vi "TEST - String to Character Array.vi"(8 "error in (no error)":errorcluster) -> (0 "error out":errorcluster, 2 "Pass":bool)   [LabVIEW 2009]
panel:
  out "Expected Result":string[](array[string])
  out "Result":string[](array[string])
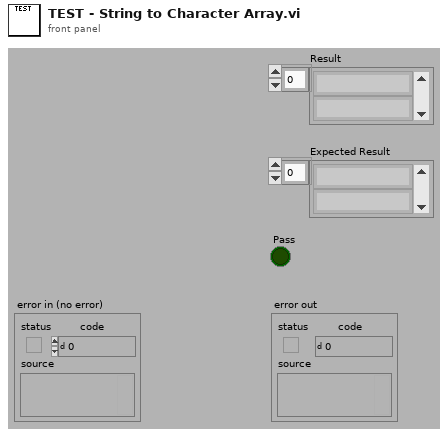
[diagram p1: front panel]
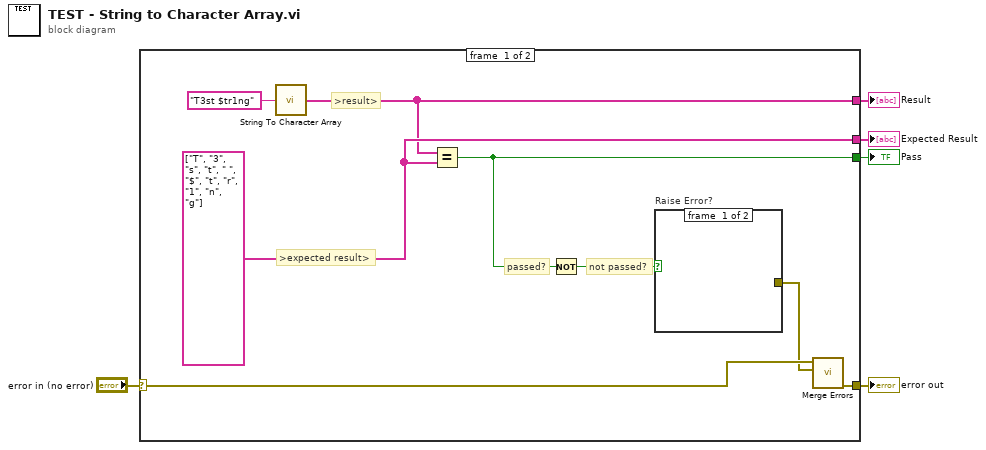
[diagram p0: block diagram]
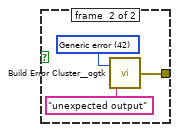
[diagram p2: hidden frame]
diagram:
  n1 = case shown="No Error" "error in (no error)" {
    selector: "error in (no error)" -> [w13 w17]
    tunnel: [w11 _] -> w5
    tunnel: [w12 w17] -> w3
    tunnel: [w6 _] -> w2
    tunnel: [w8 _] -> w1
    frame #0 {
      w8 = string[] ["T", "3", "s", "t", " ", "$", "t", "r", "1", "n", "g"] ("Character Array")
      # ">result>"
      # ">expected result>"
      # "not passed?"
      # "passed?"
      n2 = call "String To Character Array.vi"("Input String"="T3st $tr1ng") -> ("Character Array"=w6:string[])
      n3 = Equal?(x=w6, y=w8) -> (x = y?=w11:bool)
      n4 = Not(x=w11) -> (.not. x?=w9:bool)
      n5 = case "Raise Error?" shown="True" w9 {
        tunnel: [_ w14] -> w10
        frame #0 {
        }
        frame #1 {
          w15 = 42 items=["No error", "Argument error", "Memory is full", "Out of zone", "End of file", "File already open", "Generic file I/O error", "File not found", "File permission error", "Disk is full", "Duplicate path", "Too many files open", "System feature not enabled", "Resource file not found", "Cannot add resource", "Resource not found", "Image not found", "Image memory error", "Pen does not exist", "Config type invalid", "Config token not found", "Config parse error", "Config memory error", "Bad external code format", "Bad external code offset", "External code not present", "Null window", "Destroy window error", "Null menu", "Print aborted", "Bad print record", "Print driver error", "Windows error during printing", "Memory error during printing", "Print dialog error", "Generic print error", "Invalid device refnum", "Device not found", "Device parameter error", "Device unit error", "Cannot open device", "Device call aborted", "Generic error", "Cancelled by user", "Object ID too low", "Object ID too high", "Object not in heap", "Unknown heap", "Unknown object (invalid DefProc)", "Unknown object (DefProc not in table)", "Message out of range", "Invalid (null) method", "Unknown message", "Manager call not supported", "Bad address", "Network operation in progress", "Network operation timed out", "Connection is busy", "Network attribute not supported", "Network error", "Address in use", "System out of memory", "Connection aborted", "Connection refused", "Not connected", "Already connected", "Connection closed", "Initialization error (interapplication manager)", "Bad occurrence", "Wait on unbound occurrence handler", "Occurrence queue overflow", "Datalog type conflict", "Unused", "Unrecognized type (interapplication manager)", "Memory corrupt", "Failed to make temporary DLL", "Old CIN version", "Drag socket not found", "Failed to load drop-object", "Failed to register OLE object", "Failed to release OLE object", "Format specifier type mismatch", "Unknown format specifier", "Too few format specifiers", "Too many format specifiers", "Scan failed", "Newer CIN version", "Error converting to variant", "Runtime menu error", "Password tampered", "Variant attribute not found", "Incompatible variant data type", "Event data is not available", "Event Store is not present", "Occurrence is not found", "Event Queue is not created", "Event info is not available", "Refnum passed is NULL", "Error retrieving Class GUID", "Error retrieving CoClass GUID", "Error retrieving TypeLib GUID.", "Bad built application magic bytes.", "Specific driver is different from the specific driver associated with the Logical Name.", "There is no session opened to the class driver.", "Max Error", "MAX - Error with config objects", "MAX - Error loading configuration", "MAX - Group not supported"]
          n6 = call <userlib>:"Build Error Cluster__ogtk.vi"("String to Prepend to source (\"\")"="unexpected output" ("String to Prepend to source (\"\")"), "code"=w15) -> ("error out"=w14:errorcluster)
        }
      }
      n7 = call <vilib>:"Merge Errors.vi"("error in 2 (no error)"=w10, "error in 1 (no error)"=w13) -> ("error out"=w12:errorcluster)  [unwired: 5 in]
    }
    frame #1 {
    }
  }
  "Pass" <- w5
  "error out" <- w3
  "Result" <- w2
  "Expected Result" <- w1
